vi "ArraysExample_ND.vi"() -> ()   [LabVIEW 2020]
doc: "Example of N-Dimension arrays and related functions. Comments in polish language."
uses:
  <vilib>/numeric/Random Number (Range) U64.vi
  <vilib>/numeric/sub_Random U32.vi
panel:
  out "Array":u64[](array[numeric])
  out "Tablica 10 transponowana":dbl[][](array[numeric])
  in  "Tablica 10":dbl[][](array[numeric])=[[1.0, 2.0, 3.0, 4.0, 5.0], [11.0, 12.0, 13.0, 14.0, 15.0], [21.0, 22.0, 23.0, 24.0, 25.0]]
  out "Zbudowana tablica":dbl[][](array[numeric])
  out "Wybrana tablica":dbl[](array[numeric])
  out "Tablica rozmiarów":i32[](array[numeric])
  in  "Tablica 9":dbl[](array[numeric])=[6.0, 6.0, 6.0, 6.0, 6.0]
  in  "Tablica 8":dbl[](array[numeric])=[3.0, 3.0, 3.0, 3.0, 3.0]
  out "Wybrany element":dbl
  in  "Tablica 6":dbl[][](array[numeric])=[[11.0, 12.0, 13.0, 14.0, 15.0], [21.0, 22.0, 23.0, 24.0, 25.0]]
  out "Tablica programowa":dbl[][](array[numeric])
  in  "Tablica 5":dbl[][][](array[numeric])=[[[3.0, 3.0, 3.0, 3.0, 3.0], [4.0, 4.0, 4.0, 4.0, 4.0]]]
  out "Wynik tablic 1":dbl[][](array[numeric])=[[3.0, 4.0, 5.0, 6.0, 7.0], [3.0, 4.0, 5.0, 6.0, 8.0]]
  in  "Tablica 2":dbl[][](array[numeric])=[[2.0, 2.0, 2.0, 2.0, 2.0], [2.0, 2.0, 2.0, 2.0, 2.0]]
  in  "Tablica 1":dbl[][](array[numeric])=[[1.0, 2.0, 3.0, 4.0, 5.0], [1.0, 2.0, 3.0, 4.0, 6.0]]
  in  "Przykładowa tablica":dbl[][][](array[numeric])=[[[0.0, 0.0, 0.0, 0.0, 0.0], [0.0, 0.0, 0.0, 0.0, 0.0], [0.0, 0.0, 0.0, 0.0, 0.0], [0.0, 0.0, 0.0, 0.0, 4.0]], [[0.0, 0.0, 0.0, 1.0, 0.0], [0.0, 21.0, 0.0, 0.0, 0.0], [0.0, 0.0, 0.0, 0.0, 0.0], [0.0, 12.0, 0.0, 0.0, 0.0]]]
  # "1. Stworzenie najprostszej tablicy liczb i podstawowe parametry tablicy"
  # "2. Działania arymetyczne/logiczne na tablicach"
  # "3. Przegląd funkcji z palety Arrays"
  # "Array size -rozmiar tablicy"
  # "Initialize array-programowe tworzenie tablicy"
  # "Index array-pobranie wartości konkretnego elementu z tablicy"
  # "Build array - budowanie tablic wielowymiarowych"
  # "Transpose array - transponowanie tablicy 2 wymiarowej"
  # "4. Pętle i tablice"
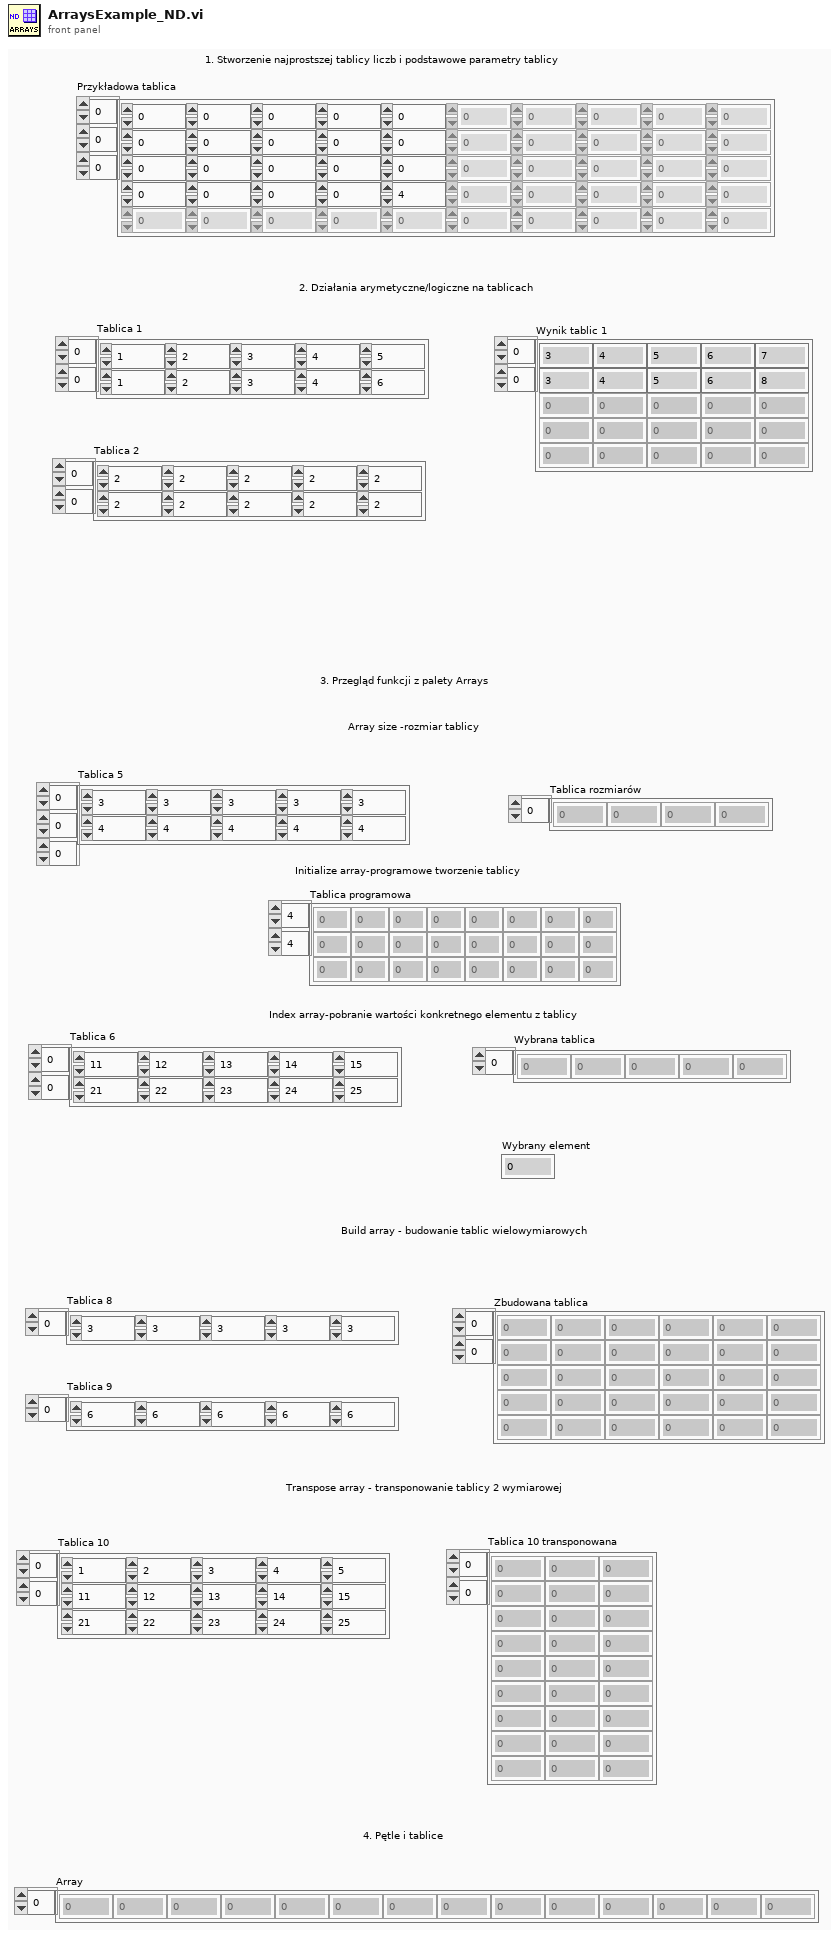
[diagram p1: front panel]
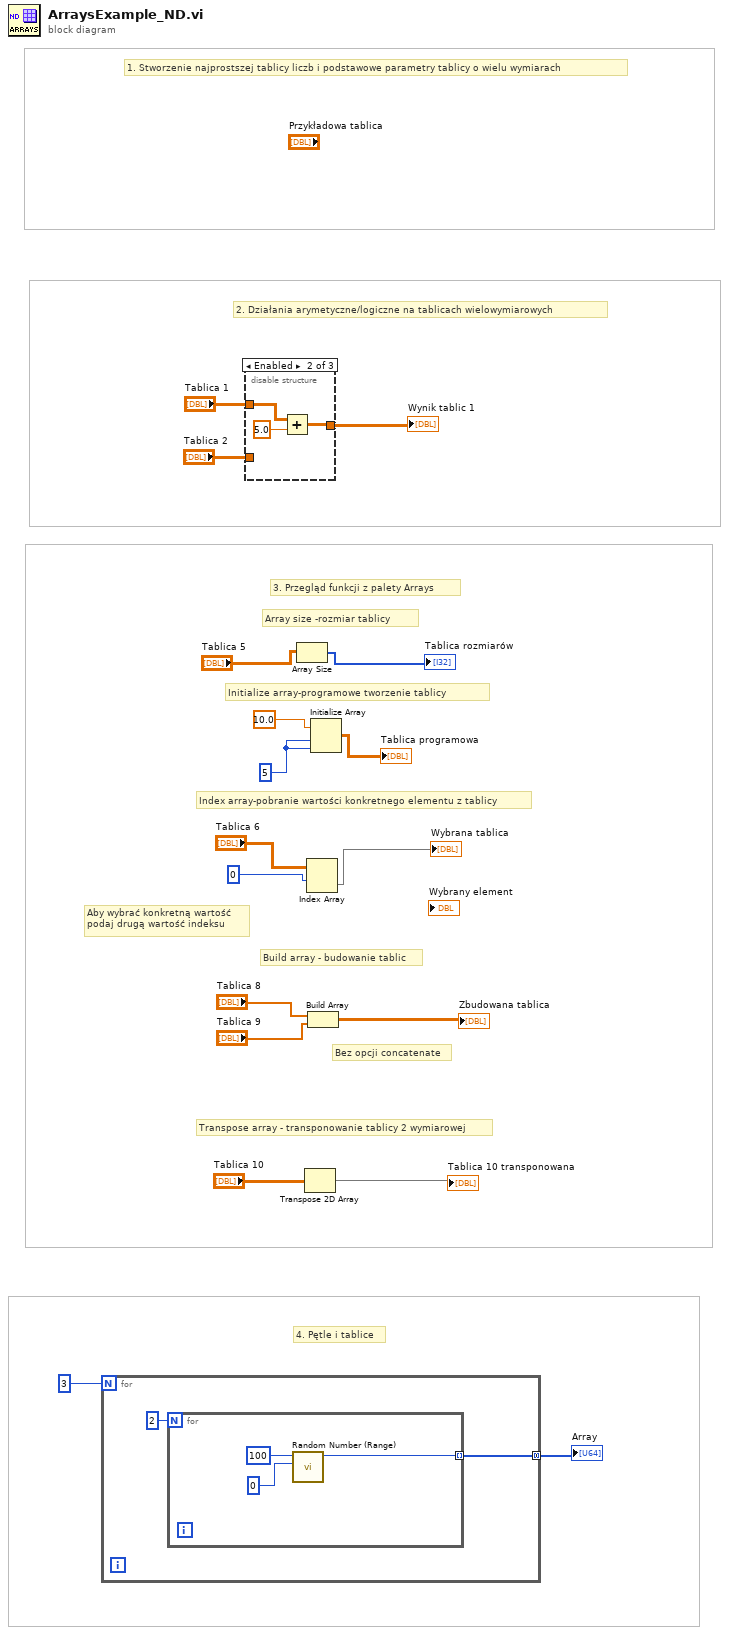
[diagram p0: block diagram]
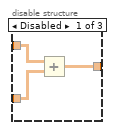
[diagram p2: hidden frame]
diagram:
  w11 = 5 ("dimension size")
  # "Bez opcji concatenate"
  # "Aby wybrać konkretną wartość\npodaj drugą wartość indeksu"
  # "Transpose array - transponowanie tablicy 2 wymiarowej"
  # "4. Pętle i tablice"
  # "Build array - budowanie tablic"
  # "Index array-pobranie wartości konkretnego elementu z tablicy"
  # "Initialize array-programowe tworzenie tablicy"
  # "Array size -rozmiar tablicy"
  # "3. Przegląd funkcji z palety Arrays"
  # "2. Działania arymetyczne/logiczne na tablicach wielowymiarowych"
  # "1. Stworzenie najprostszej tablicy liczb i podstawowe parametry tablicy o wielu wymiarach"
  n1 = for {
    N: 3 -> [_]
    tunnel: [w19] -> w1 mode=concatenating
    n2 = for {
      N: 2 -> [_]
      tunnel: [w21] -> w19 mode=indexing
      n3 = call-poly <vilib>:"Random Number (Range).vi"("lower bound (0)"=u64 0, "upper bound (100)"=u64 100) -> ("number"=w21:u64)  [unwired: 9 in]
    }
  }
  "Array" <- w1
  n4 = disable-structure shown="Enabled" {
    disable-tunnel: "Tablica 1" -> [w26 w28 _]
    disable-tunnel: "Tablica 2" -> [w25 _ _]
    disable-tunnel: [w24 w27 _] -> w15
    frame Disabled {
      n5 = Add(x=w26, y=w25) -> (x+y=w24:dbl[][])
    }
    frame Enabled {
      n6 = Add(x=w28, y=5.0) -> (x+y=w27:dbl[][])
    }
    frame Disabled {
    }
  }
  "Wynik tablic 1" <- w15
  n7 = Array Size(array="Tablica 5") -> (size(s)=→"Tablica rozmiarów":i32[])
  n8 = Transpose 2D Array(2D array="Tablica 10") -> (transposed array=→"Tablica 10 transponowana":dbl[][])
  n9 = Index Array(array="Tablica 6", index (row)=0) -> (element=→"Wybrana tablica":dbl[])  [unwired: 1 in]
  n10 = Build Array("Tablica 8", "Tablica 9") -> (→"Zbudowana tablica":dbl[][])
  n11 = Initialize Array(10.0, w11, w11) -> (→"Tablica programowa":dbl[][])
